vi "Open Joysticks.vi"(8 "error in (no error)":errorcluster) -> (0 "error out":errorcluster)   [LabVIEW 2018]
uses:
  <vilib>/Rock Robotics/WPI/Joystick/WPI_JoystickDeviceEnum.ctl
  TypeDefs/typedef_enum_Refnums.ctl
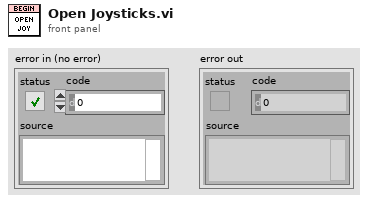
[diagram p1: front panel]
types:
  T1 = typedef "typedef_enum_Refnums.ctl" = enum16{"Ball_Encoder", "Ball_Motor", "Camera", "Linefollow_3", "Linefollow_2", "Linefollow_1", "Gyro", "Hatch_Solenoid", "Climb_Back_Solenoid", "Arm_Encoder", "Arm_Motor", "Lift_Encoder", "Drive", "Drive_Motor_R", "Drive_Motor_L", "Drive_Encoder_R", "Drive_Encoder_L", "Joy_R", "Joy_L", "Wrist_Motor", "Wrist_Encoder", "Climb_Front_Encoder", "Climb_Front_Motor"}
  T2 = typedef "WPI_JoystickDeviceEnum.ctl" = enum16{"USB 0", "USB 1", "USB 2", "USB 3", "USB 4", "USB 5"}
  T3 = typedef "WPI_JoystickDevRef.ctl" = cluster{"Device":T2}
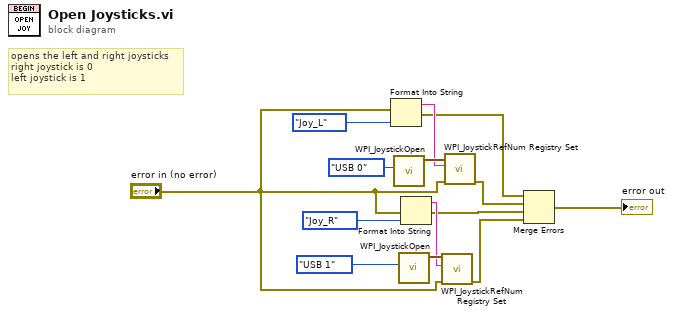
[diagram p0: block diagram]
diagram:
  # "opens the left and right joysticks\nright joystick is 0 \nleft joystick is 1"
  n1 = Format Into String(error in="error in (no error)", typedef_enum_Refnums."Joy_L" ("RefNums")) -> (resulting string=w9:string, error out=w6:errorcluster)  [unwired: 2 in]
  n2 = call <vilib>:"WPI_JoystickOpen.vi"("JoystickDevice"=WPI_JoystickDeviceEnum."USB 0") -> ("JoystickDevRef"=w12:T3)  [unwired: 10 in]
  n3 = call <vilib>:"WPI_JoystickOpen.vi"("JoystickDevice"=WPI_JoystickDeviceEnum."USB 1") -> ("JoystickDevRef"=w11:T3)  [unwired: 10 in]
  n4 = Format Into String(error in="error in (no error)", typedef_enum_Refnums."Joy_R" ("RefNums")) -> (resulting string=w7:string, error out=w4:errorcluster)  [unwired: 2 in]
  n5 = call <vilib>:"WPI_JoystickRefNum Registry Set.vi"("error in (no error)"="error in (no error)", "refnum name"=w7, "JoystickDevRef"=w11) -> ("error out"=w2:errorcluster)  [unwired: 7 in, 1 out]
  n6 = call <vilib>:"WPI_JoystickRefNum Registry Set.vi"("error in (no error)"="error in (no error)", "refnum name"=w9, "JoystickDevRef"=w12) -> ("error out"=w5:errorcluster)  [unwired: 7 in, 1 out]
  n7 = Merge Errors(w6, w5, w4, w2) -> (→"error out":errorcluster)
